vi "赋值.vi"(7 "This VI":refnum<vi>, 8 "temp":string[](array[string]), 9 "fengshan":string[](array[string]), 10 "机箱index":i32, 11 "主控选项卡":refnum<vi>) -> ()   [LabVIEW 2015]
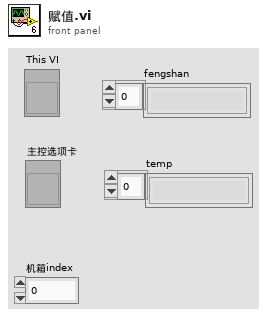
[diagram p1: front panel]
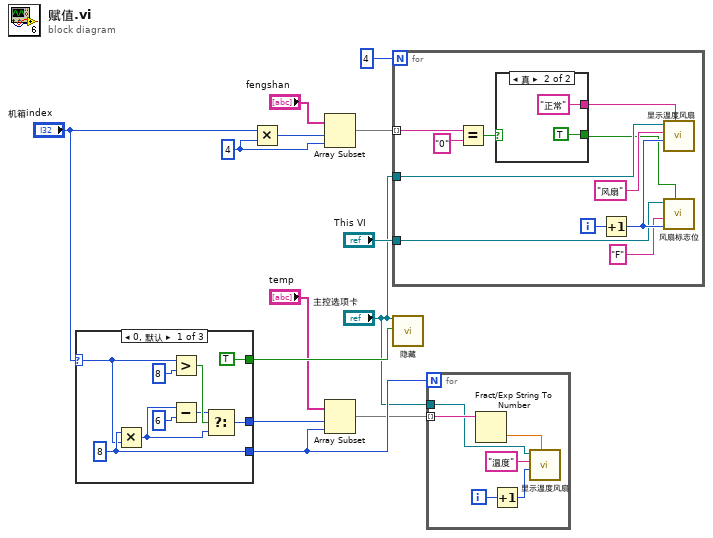
[diagram p0: block diagram]
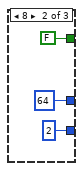
[diagram p2: hidden frame]
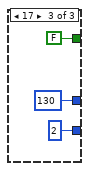
[diagram p3: hidden frame]
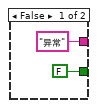
[diagram p4: hidden frame]
diagram:
  w10 = 4 ("y")
  n1 = case shown="0, 默认" "机箱index" {
    selector: "机箱index" -> [w21 _ _]
    tunnel: [w22 2 2] -> w7
    tunnel: [w15 64 130] -> w6
    tunnel: [TRUE FALSE FALSE] -> w4
    frame 0, Default {
      w22 = 8
      n2 = Multiply(x=w22, y=w21) -> (x*y=w18:i32)
      n3 = Greater?(x=w21, y=8) -> (0:w19:bool)
      n4 = Subtract(x=w18, y=6) -> (x-y=w16:i32)
      n5 = Select(t=w16, s=w19, f=w18) -> (s? t:f=w15:i32)
    }
    frame 8 {
    }
    frame 17 {
    }
  }
  n6 = Multiply(x="机箱index", y=w10) -> (x*y=w9:i32)
  n7 = Array Subset(array="fengshan", index=w9, length=w10) -> (w8:string[])
  n8 = Array Subset(array="temp", index=w6, length=w7) -> (w5:string[])
  n9 = for {
    N: 4 -> [_]
    tunnel: w8 -> [w36] mode=indexing
    tunnel: "主控选项卡" -> [w31]
    tunnel: "This VI" -> [w29]
    i -> [w38]
    n10 = Equal?(x=w36, y="0") -> (x = y?=w35:bool)
    n11 = case shown="真" w35 {
      tunnel: ["异常" "正常"] -> w34
      tunnel: [FALSE TRUE] -> w30
      frame False {
      }
      frame True {
      }
    }
    n12 = Increment(x=w38) -> (x+1=w33:i32)
    n13 = call "显示温度风扇.vi"("Value"=w34, "索引"=w33, "类别"="风扇", "Tab Control"=w31) -> ()  [unwired: 8 in]
    n14 = call "风扇标志位.vi"("Value"=w30, "索引"=w33, "类别"="F", "vi refnum"=w29) -> ()  [unwired: 8 in]
  }
  n15 = call "隐藏.vi"("Tab Control"="主控选项卡", "visible"=w4) -> ()  [unwired: 18 in]
  n16 = for {
    N: w7 -> [_]
    tunnel: w5 -> [w46] mode=indexing
    tunnel: "主控选项卡" -> [w44]
    i -> [w48]
    n17 = Fract/Exp String To Number(string=w46) -> (number=w45:dbl)  [unwired: 3 in, 1 out]
    n18 = Increment(x=w48) -> (x+1=w47:i32)
    n19 = call "显示温度风扇.vi"("Value"=w45, "索引"=w47, "类别"="温度", "Tab Control"=w44) -> ()  [unwired: 8 in]
  }
